vi "Close Report File.vi"(8 "error in (no error)":errorcluster, 11 "XML Report In":refnum<class "XML Report.lvclass">) -> (0 "error out":errorcluster, 2 "Report Path":path)   [LabVIEW 2020, in "Reports.lvlib" / "XML Report.lvclass"]
uses:
  XML Report.lvclass
  XML Report.lvclass/XML Report.ctl
  <vilib>/xml/Close Reference(Node).vi
  <vilib>/xml/NI_XML.lvlib
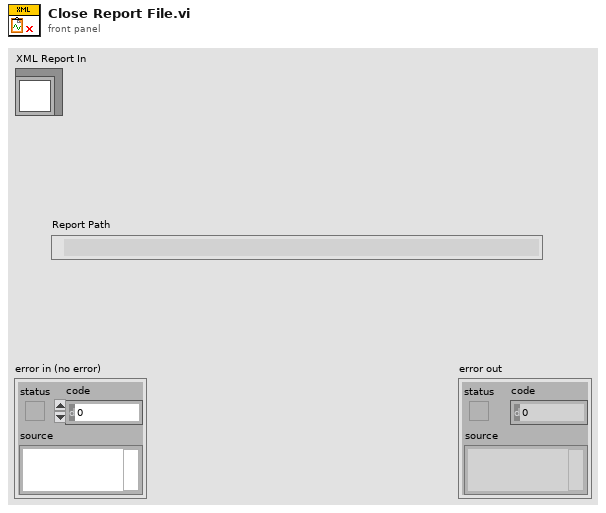
[diagram p1: front panel]
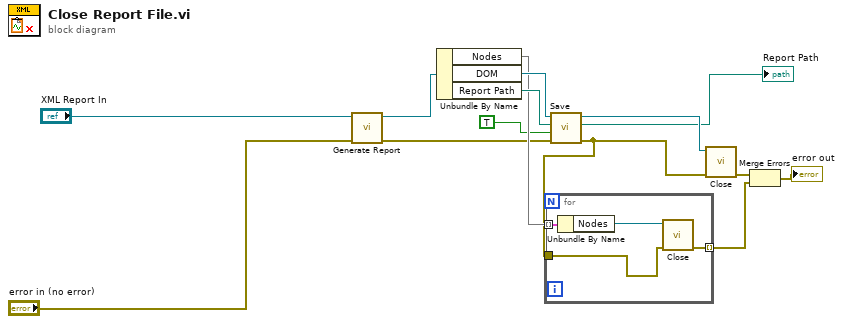
[diagram p0: block diagram]
diagram:
  n1 = call "Generate Report.vi"("error in (no error)"="error in (no error)", "XML Report In"="XML Report In") -> ("error out"=w7:errorcluster, "XML Report Out"=w6:refnum<class "XML Report.lvclass">)  [unwired: 8 in]
  n2 = Unbundle By Name(w6) -> ("Nodes"=w10:map{string, refnum<k20>}, "DOM"=w14:refnum<k20>, "Report Path"=w11:path)
  n3 = call <vilib>:"Save.vi"("error in (no error)"=w7, "overwrite file (True)"=TRUE, "XML file path"=w11, "DOM document in"=w14) -> ("error out"=w2:errorcluster, "XML file path out"=→"Report Path":path, "DOM document out"=w13:refnum<k20>)  [unwired: 5 in]
  n4 = for {
    tunnel: w10 -> [w18] mode=indexing
    tunnel: [w16] -> w9 mode=indexing
    tunnel: w2 -> [w15]
    n5 = Unbundle By Name(w18) -> ("Nodes"=w17:refnum<k20>)
    n6 = call-poly <vilib>:"Close.vi"("error in (no error)"=w15, "node"=w17) -> ("error out"=w16:errorcluster)  [unwired: 7 in]
  }
  n7 = call-poly <vilib>:"Close.vi"("error in (no error)"=w2, "node"=w13) -> ("error out"=w8:errorcluster)  [unwired: 7 in]
  n8 = Merge Errors(w8, w9) -> (→"error out":errorcluster)
